vi "_sortItemsByColumnIndex.vi"(6 "times":i32, 8 "Indices":i32[](array[numeric]), 9 "DataPlugin information":T1[](array[typedef]), 10 "column Index":i32, 11 "Items in":string[][](array[string])) -> (0 "times out":i32, 1 "Indices out":i32[](array[numeric]), 2 "DataPlugin information out":T1[](array[typedef]), 3 "Items out":string[][](array[string]))   [LabVIEW 2017]
uses:
  <vilib>/Platform/storage/utility/DataPluginSynchronization/_DataPluginInfo.ctl
  <vilib>/Platform/storage/utility/DataPluginSynchronization/_localizeDataPluginMessageEnum.ctl
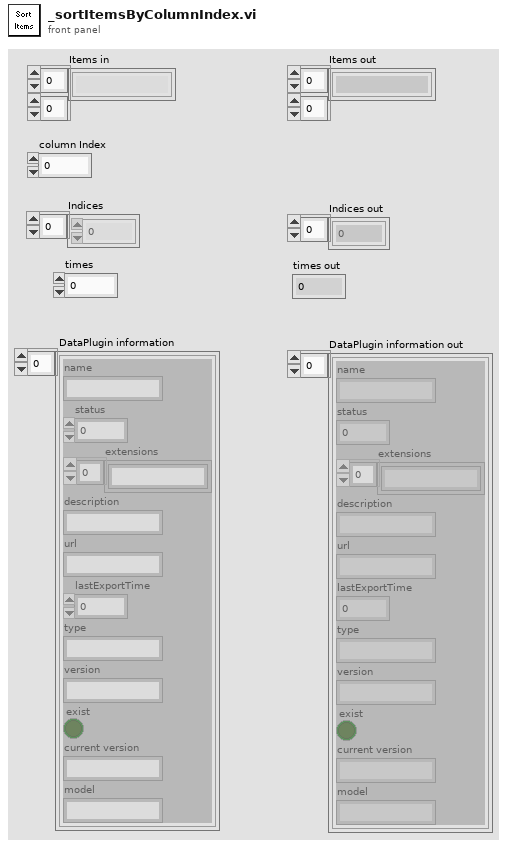
[diagram p1: front panel]
types:
  T1 = typedef "_DataPluginInfo.ctl" = cluster{"name":string, "status":u32, "extensions":string[], "description":string, "url":string, "lastExportTime":i64, "type":string, "version":string, "exist":bool, "current version":string, "model":string}
  T2 = typedef "_localizeDataPluginMessageEnum.ctl" = enum16{"Installed", "Not Installed", "Updates Available", "Latest version:", "Double click the \"Description\" cell.", "Install/Update DataPlugins", "Offline: ", "Please ensure that your network connection is working.", "No DataPlugins can be updated.", "Loading DataPlugins from ni.com/dataplugins", "Acquiring and installing ", "Install", "Update", "Succeed", "Failed", " Installation successful.", "Include *. to search for a file extension", "Current version:", " Installation failed.", "Installing update", "Update successful.", "Update failed.", "Updated", "Failed to update DataPlugins."}
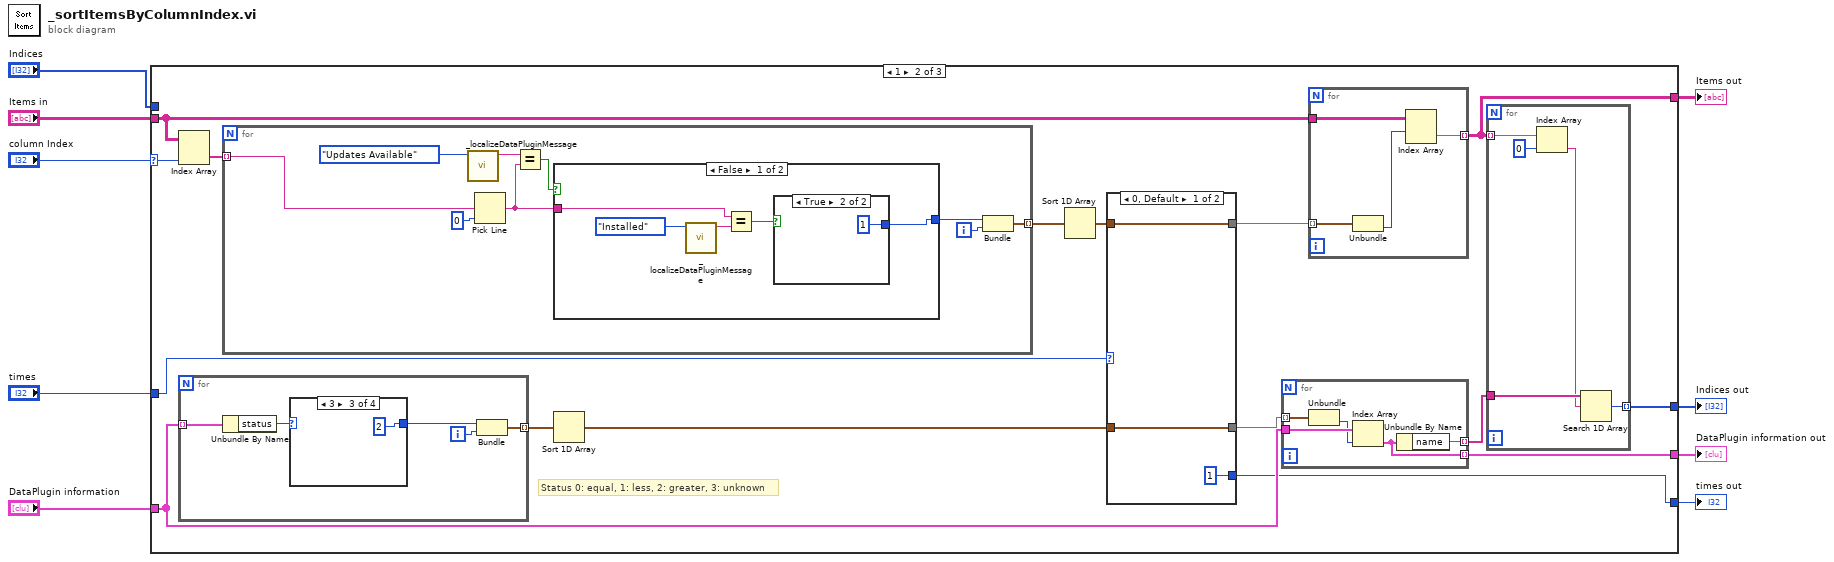
[diagram p0: block diagram]
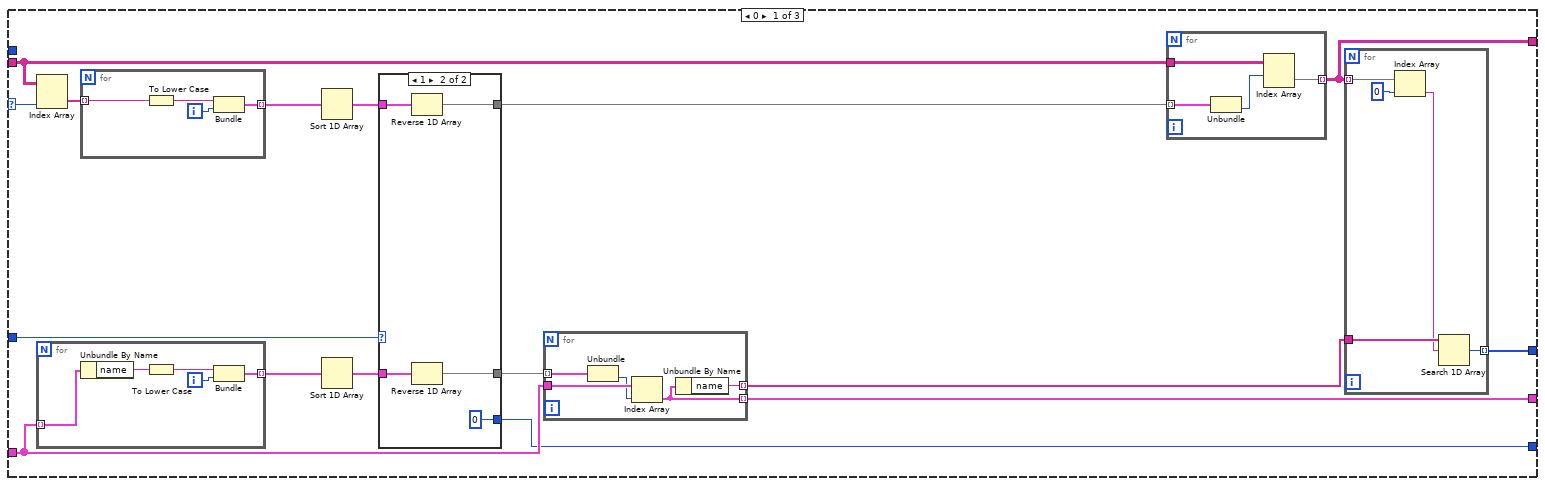
[diagram p2: hidden frame]
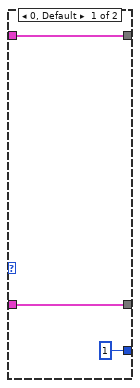
[diagram p3: hidden frame]
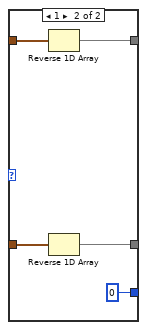
[diagram p4: hidden frame]
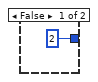
[diagram p5: hidden frame]
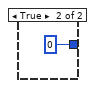
[diagram p6: hidden frame]
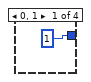
[diagram p7: hidden frame]
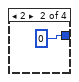
[diagram p8: hidden frame]
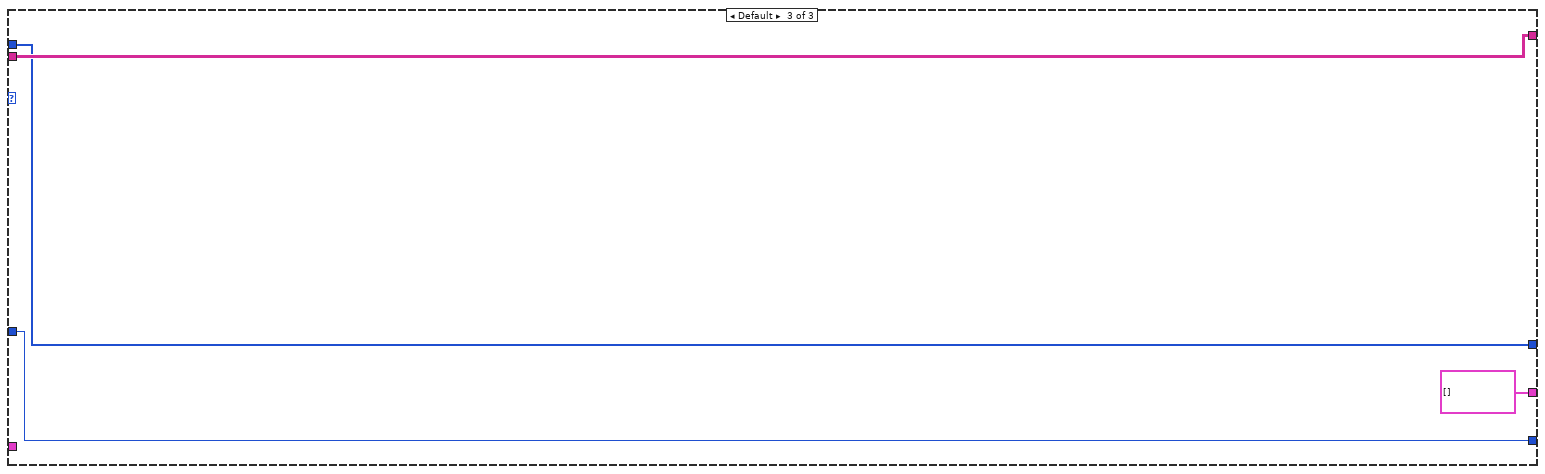
[diagram p10: hidden frame]
diagram:
  n1 = case shown="1" "column Index" {
    selector: "column Index" -> [w24 w68 _]
    tunnel: "DataPlugin information" -> [w20 w63 _]
    tunnel: [w22 w72 T1[] []] -> w9
    tunnel: "Items in" -> [w23 w69 w123]
    tunnel: [w18 w67 w123] -> w6
    tunnel: "Indices" -> [_ _ w122]
    tunnel: [w21 w65 w122] -> w4
    tunnel: "times" -> [w14 w62 w121]
    tunnel: [w10 w61 w121] -> w2
    frame 0 {
      n2 = Index Array(array=w23, index (col)=w24) -> (element=w19:string[])  [unwired: 1 in]
      n3 = for {
        tunnel: w20 -> [w54] mode=indexing
        tunnel: [w55] -> w25 mode=indexing
        i -> [w56]
        n4 = Unbundle By Name(w54) -> ("name"=w53:string)
        n5 = To Lower Case(string=w53) -> (all lower case string=w52:string)
        n6 = Bundle(w52, w56) -> (w55:cluster{string, i32})  [unwired: 1 in]
      }
      n7 = for {
        tunnel: w19 -> [w49] mode=indexing
        tunnel: [w50] -> w17 mode=indexing
        i -> [w51]
        n8 = To Lower Case(string=w49) -> (all lower case string=w48:string)
        n9 = Bundle(w48, w51) -> (w50:cluster{string, i32})  [unwired: 1 in]
      }
      n10 = Sort 1D Array(array=w17) -> (sorted array=w15:cluster{string, i32}[])
      n11 = Sort 1D Array(array=w25) -> (sorted array=w12:cluster{string, i32}[])
      n12 = case shown="1" w14 {
        tunnel: [w33 w38] -> w16
        tunnel: w15 -> [w33 w37]
        tunnel: w12 -> [w32 w36]
        tunnel: [w32 w35] -> w11
        tunnel: [1 ("times") 0 ("times")] -> w10
        frame 0, Default {
        }
        frame 1 {
          n13 = Reverse 1D Array(array=w37) -> (reversed array=w38:cluster{string, i32}[])
          n14 = Reverse 1D Array(array=w36) -> (reversed array=w35:cluster{string, i32}[])
        }
      }
      n15 = for {
        tunnel: w11 -> [w30] mode=indexing
        tunnel: [w27] -> w22 mode=indexing
        tunnel: w20 -> [w29]
        tunnel: [w26] -> w13 mode=indexing
        n16 = Unbundle(w30) -> (w28:i32)  [unwired: 1 out]
        n17 = Index Array(array=w29, index=w28) -> (element=w27:T1)
        n18 = Unbundle By Name(w27) -> ("name"=w26:string)
      }
      n19 = for {
        tunnel: w16 -> [w42] mode=indexing
        tunnel: [w40] -> w18 mode=indexing
        tunnel: w23 -> [w41]
        n20 = Unbundle(w42) -> (w39:i32)  [unwired: 1 out]
        n21 = Index Array(array=w41, index (row)=w39) -> (element=w40:string[])  [unwired: 1 in]
      }
      n22 = for {
        tunnel: w18 -> [w47] mode=indexing
        tunnel: w13 -> [w45]
        tunnel: [w43] -> w21 mode=indexing
        n23 = Index Array(array=w47, index=0) -> (element=w44:string)
        n24 = Search 1D Array(1D array=w45, element=w44) -> (index of element=w43:i32)  [unwired: 1 in]
      }
    }
    frame 1 {
      # "Status 0: equal, 1: less, 2: greater, 3: unknown"
      n25 = Index Array(array=w69, index (col)=w68) -> (element=w71:string[])  [unwired: 1 in]
      n26 = for {
        tunnel: w63 -> [w116] mode=indexing
        tunnel: [w115] -> w64 mode=indexing
        i -> [w112]
        n27 = Unbundle By Name(w116) -> ("status"=w114:u32)
        n28 = case shown="3" w114 {
          selector: w114 -> [_ _ _ w120]
          tunnel: [u32 1 ("status") u32 0 ("status") u32 2 ("status") w120] -> w113
          frame 0, 1 {
          }
          frame 2 {
          }
          frame 3 {
          }
          frame Default {
          }
        }
        n29 = Bundle("status"=w113, w112) -> (w115:cluster{"status":u32, i32})  [unwired: 1 in]
      }
      n30 = for {
        tunnel: w71 -> [w101] mode=indexing
        tunnel: [w102] -> w70 mode=indexing
        i -> [w103]
        n31 = call <vilib>:"_localizeDataPluginMessage.vi"("message in"=_localizeDataPluginMessageEnum."Updates Available") -> ("message out"=w98:string)  [unwired: 10 in]
        n32 = Pick Line(multi-line string=w101, line index=0) -> (output string=w95:string)  [unwired: 1 in]
        n33 = Equal?(x=w98, y=w95) -> (x = y?=w97:bool)
        n34 = case shown="False" w97 {
          tunnel: [w104 u32 0 ("status")] -> w96
          tunnel: w95 -> [w107 _]
          frame False {
            n35 = call <vilib>:"_localizeDataPluginMessage.vi"("message in"=_localizeDataPluginMessageEnum."Installed") -> ("message out"=w106:string)  [unwired: 10 in]
            n36 = Equal?(x=w107, y=w106) -> (x = y?=w105:bool)
            n37 = case shown="True" w105 {
              tunnel: [u32 2 ("status") u32 1 ("status")] -> w104
              frame False {
              }
              frame True {
              }
            }
          }
          frame True {
          }
        }
        n38 = Bundle("status"=w96, w103) -> (w102:cluster{"status":u32, i32})  [unwired: 1 in]
      }
      n39 = Sort 1D Array(array=w64) -> (sorted array=w58:cluster{"status":u32, i32}[])
      n40 = Sort 1D Array(array=w70) -> (sorted array=w60:cluster{"status":u32, i32}[])
      n41 = case shown="0, Default" w62 {
        tunnel: [1 ("times") 0 ("times")] -> w61
        tunnel: w60 -> [w74 w79]
        tunnel: [w74 w78] -> w59
        tunnel: w58 -> [w73 w77]
        tunnel: [w73 w76] -> w57
        frame 0, Default {
        }
        frame 1 {
          n42 = Reverse 1D Array(array=w79) -> (reversed array=w78:cluster{"status":u32, i32}[])
          n43 = Reverse 1D Array(array=w77) -> (reversed array=w76:cluster{"status":u32, i32}[])
        }
      }
      n44 = for {
        tunnel: w57 -> [w85] mode=indexing
        tunnel: [w82] -> w72 mode=indexing
        tunnel: [w81] -> w66 mode=indexing
        tunnel: w63 -> [w84]
        n45 = Unbundle(w85) -> (w83:i32)  [unwired: 1 out]
        n46 = Index Array(array=w84, index=w83) -> (element=w82:T1)
        n47 = Unbundle By Name(w82) -> ("name"=w81:string)
      }
      n48 = for {
        tunnel: w59 -> [w89] mode=indexing
        tunnel: [w87] -> w67 mode=indexing
        tunnel: w69 -> [w88]
        n49 = Unbundle(w89) -> (w86:i32)  [unwired: 1 out]
        n50 = Index Array(array=w88, index (row)=w86) -> (element=w87:string[])  [unwired: 1 in]
      }
      n51 = for {
        tunnel: w67 -> [w94] mode=indexing
        tunnel: w66 -> [w92]
        tunnel: [w91] -> w65 mode=indexing
        n52 = Index Array(array=w94, index=0) -> (element=w90:string)
        n53 = Search 1D Array(1D array=w92, element=w90) -> (index of element=w91:i32)  [unwired: 1 in]
      }
    }
    frame Default {
    }
  }
  "Items out" <- w6
  "DataPlugin information out" <- w9
  "Indices out" <- w4
  "times out" <- w2
